vi "Read Dashboard Variables.vi"() -> ()   [LabVIEW 2018]
uses:
  <vilib>/Rock Robotics/Network Tables/NT Read Number.vi
  Framework/Robot Global Data.vi
panel:
  out "Hatch Mover Duration":dbl=3.0
  out "Hatch Mover Setpoint":dbl=1.0
  out "SlowModeSettings":i32=2
  out "MaxSpeedSlow":dbl=0.4
  out "SlowRate":dbl=1.0
  out "MaxTurnSlow":dbl=0.55
  out "MaxTurnRateSlow":dbl=20.0
  out "Cargo Stop Current":dbl=10.0
  out "Cargo Hold Duration":dbl=1.0
  out "Cheezy Drive Mode":u32=2
  out "Cargo Setpoint":dbl=1.0 min=0.0 max=1.0 step=0.1
  out "Elevator Duration":dbl
  out "Elevator Setpoint":dbl=1.0 min=0.0 max=1.0 step=0.1
  out "Pivot Right Setpoint":dbl=0.3 min=0.0 max=1.0 step=0.1
  out "Pivot Left Setpoint":dbl=0.3 min=0.0 max=1.0 step=0.1
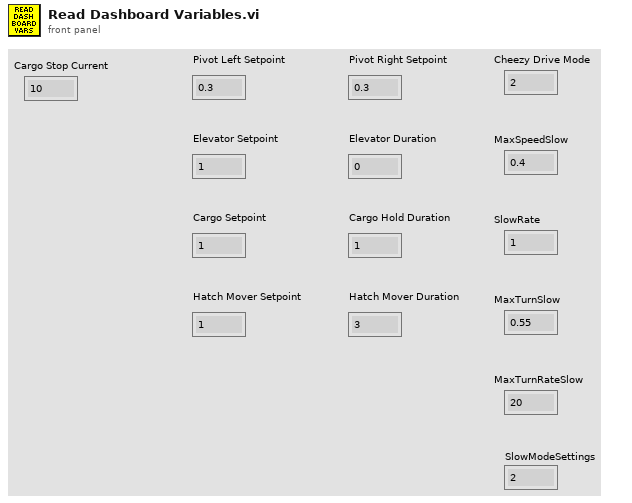
[diagram p1: front panel]
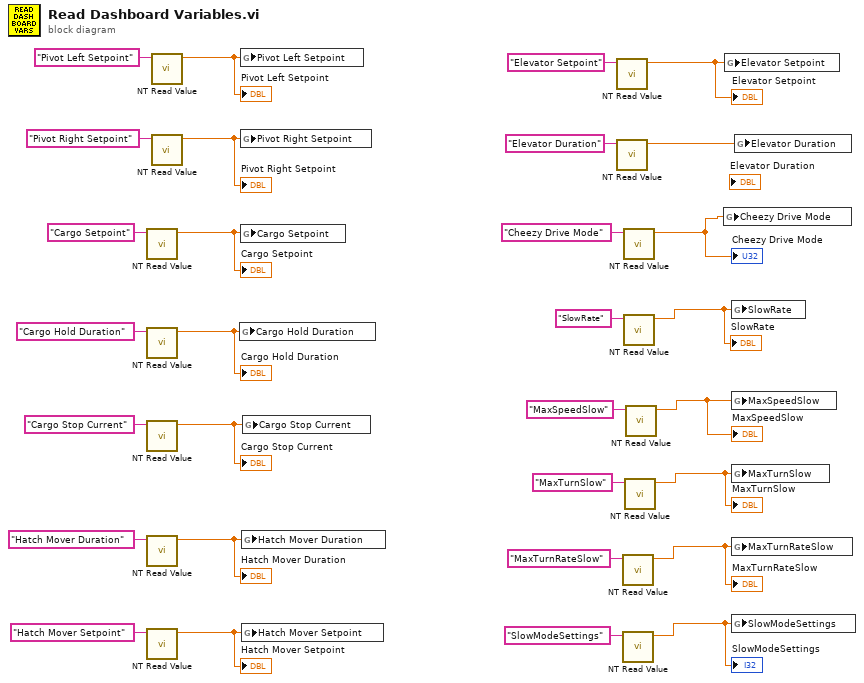
[diagram p0: block diagram]
diagram:
  n1 = call-poly <vilib>:"NT Read Value.vi"("Name"="Cargo Setpoint") -> ("Numeric"=w12:dbl)  [unwired: 9 in, 1 out]
  "Cargo Setpoint" <- w12
  n2 = call-poly <vilib>:"NT Read Value.vi"("Name"="Cargo Hold Duration") -> ("Numeric"=w11:dbl)  [unwired: 9 in, 1 out]
  "Cargo Hold Duration" <- w11
  n3 = call-poly <vilib>:"NT Read Value.vi"("Name"="Cargo Stop Current") -> ("Numeric"=w10:dbl)  [unwired: 9 in, 1 out]
  "Cargo Stop Current" <- w10
  n4 = call-poly <vilib>:"NT Read Value.vi"("Name"="Hatch Mover Duration") -> ("Numeric"=w9:dbl)  [unwired: 9 in, 1 out]
  "Hatch Mover Duration" <- w9
  n5 = call-poly <vilib>:"NT Read Value.vi"("Name"="Hatch Mover Setpoint") -> ("Numeric"=w8:dbl)  [unwired: 9 in, 1 out]
  "Hatch Mover Setpoint" <- w8
  n6 = call-poly <vilib>:"NT Read Value.vi"("Name"="Pivot Left Setpoint") -> ("Numeric"=w14:dbl)  [unwired: 9 in, 1 out]
  "Pivot Left Setpoint" <- w14
  n7 = call-poly <vilib>:"NT Read Value.vi"("Name"="Pivot Right Setpoint") -> ("Numeric"=w13:dbl)  [unwired: 9 in, 1 out]
  "Pivot Right Setpoint" <- w13
  n8 = global write "Robot Global Data.vi" "Cargo Hold Duration"(w11) -> ()
  n9 = global write "Robot Global Data.vi" "Pivot Left Setpoint"(w14) -> ()
  n10 = global write "Robot Global Data.vi" "Pivot Right Setpoint"(w13) -> ()
  n11 = global write "Robot Global Data.vi" "Cargo Setpoint"(w12) -> ()
  n12 = global write "Robot Global Data.vi" "Hatch Mover Duration"(w9) -> ()
  n13 = global write "Robot Global Data.vi" "Hatch Mover Setpoint"(w8) -> ()
  n14 = global write "Robot Global Data.vi" "Cargo Stop Current"(w10) -> ()
  n15 = call-poly <vilib>:"NT Read Value.vi"("Name"="Elevator Setpoint") -> ("Numeric"=w1:dbl)  [unwired: 9 in, 1 out]
  "Elevator Setpoint" <- w1
  n16 = call-poly <vilib>:"NT Read Value.vi"("Name"="Elevator Duration") -> ("Numeric"=w24:dbl)  [unwired: 9 in, 1 out]
  n17 = call-poly <vilib>:"NT Read Value.vi"("Name"="MaxTurnRateSlow") -> ("Numeric"=w3:dbl)  [unwired: 9 in, 1 out]
  "MaxTurnRateSlow" <- w3
  n18 = call-poly <vilib>:"NT Read Value.vi"("Name"="SlowModeSettings") -> ("Numeric"=w2:dbl)  [unwired: 9 in, 1 out]
  "SlowModeSettings" <- w2
  n19 = call-poly <vilib>:"NT Read Value.vi"("Name"="Cheezy Drive Mode") -> ("Numeric"=w7:dbl)  [unwired: 9 in, 1 out]
  "Cheezy Drive Mode" <- w7
  n20 = call-poly <vilib>:"NT Read Value.vi"("Name"="SlowRate") -> ("Numeric"=w6:dbl)  [unwired: 9 in, 1 out]
  "SlowRate" <- w6
  n21 = call-poly <vilib>:"NT Read Value.vi"("Name"="MaxTurnSlow") -> ("Numeric"=w4:dbl)  [unwired: 9 in, 1 out]
  "MaxTurnSlow" <- w4
  n22 = call-poly <vilib>:"NT Read Value.vi"("Name"="MaxSpeedSlow") -> ("Numeric"=w5:dbl)  [unwired: 9 in, 1 out]
  "MaxSpeedSlow" <- w5
  n23 = global write "Robot Global Data.vi" "Cheezy Drive Mode"(w7) -> ()
  n24 = global write "Robot Global Data.vi" "Elevator Setpoint"(w1) -> ()
  n25 = global write "Robot Global Data.vi" "SlowRate"(w6) -> ()
  n26 = global write "Robot Global Data.vi" "MaxSpeedSlow"(w5) -> ()
  n27 = global write "Robot Global Data.vi" "MaxTurnSlow"(w4) -> ()
  n28 = global write "Robot Global Data.vi" "MaxTurnRateSlow"(w3) -> ()
  n29 = global write "Robot Global Data.vi" "SlowModeSettings"(w2) -> ()
  n30 = global write "Robot Global Data.vi" "Elevator Duration"(w24) -> ()
